vi "DecodeOperationalSettingsPressure SubVI.vi"(3 "PressureMode":u8, 4 "PressureReference":u8, 5 "PressureUnitCode":u8) -> (0 "PressureMode Comment":string, 1 "Pressure Reference Comment":string, 2 "PressureUnitCode Comment":string)   [LabVIEW 2019]
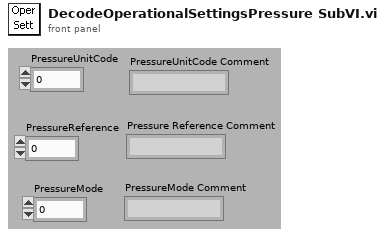
[diagram p1: front panel]
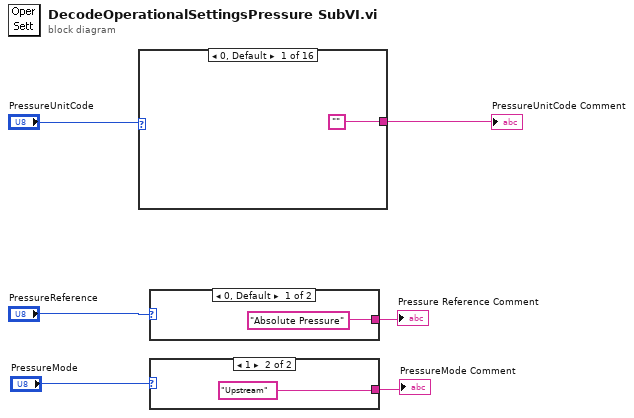
[diagram p0: block diagram]
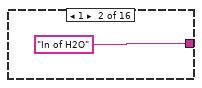
[diagram p2: hidden frame]
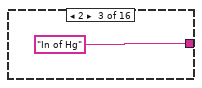
[diagram p3: hidden frame]
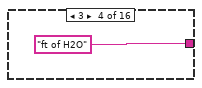
[diagram p4: hidden frame]
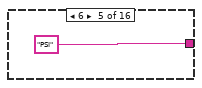
[diagram p5: hidden frame]
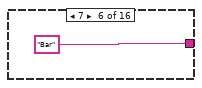
[diagram p6: hidden frame]
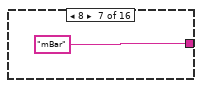
[diagram p7: hidden frame]
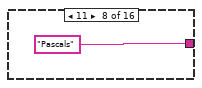
[diagram p8: hidden frame]
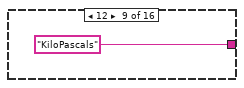
[diagram p9: hidden frame]
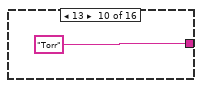
[diagram p10: hidden frame]
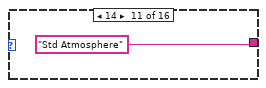
[diagram p11: hidden frame]
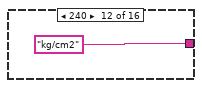
[diagram p12: hidden frame]
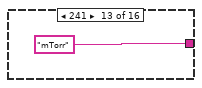
[diagram p13: hidden frame]
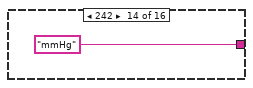
[diagram p14: hidden frame]
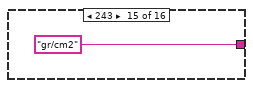
[diagram p15: hidden frame]
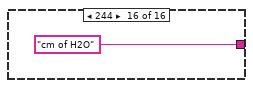
[diagram p16: hidden frame]
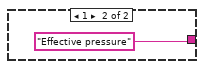
[diagram p17: hidden frame]
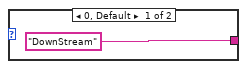
[diagram p18: hidden frame]
diagram:
  n1 = case shown="0, Default" "PressureUnitCode" {
    tunnel: ["" "In of H2O" "In of Hg" "ft of H2O" "PSI" "Bar" "mBar" "Pascals" "KiloPascals" "Torr" "Std Atmosphere" "kg/cm2" "mTorr" "mmHg" "gr/cm2" "cm of H2O"] -> w1
    frame 0, Default {
    }
    frame 1 {
    }
    frame 2 {
    }
    frame 3 {
    }
    frame 6 {
    }
    frame 7 {
    }
    frame 8 {
    }
    frame 11 {
    }
    frame 12 {
    }
    frame 13 {
    }
    frame 14 {
    }
    frame 240 {
    }
    frame 241 {
    }
    frame 242 {
    }
    frame 243 {
    }
    frame 244 {
    }
  }
  "PressureUnitCode Comment" <- w1
  n2 = case shown="0, Default" "PressureReference" {
    tunnel: ["Absolute Pressure" "Effective pressure"] -> w5
    frame 0, Default {
    }
    frame 1 {
    }
  }
  "Pressure Reference Comment" <- w5
  n3 = case shown="1" "PressureMode" {
    tunnel: ["DownStream" "Upstream"] -> w6
    frame 0, Default {
    }
    frame 1 {
    }
  }
  "PressureMode Comment" <- w6
